vi "FindSectorBox.vi"(6 "reduce pts by factor of":i32=4, 7 "Sector EndPts":T5 {"y4" format="%.2f"; "x4" format="%.2f"; "y3" format="%.2f"; "x3" format="%.2f"; "y2" format="%.2f"; "x2" format="%.2f"; "y1" format="%.2f"; "x1" format="%.2f"}, 8 "sector size":cluster{"pixels in x":i16, "pixels in y":i16}={"pixels in x"=500, "pixels in y"=400}, 9 "directory path":path, 10 "File Array":string[](array[string]), 11 "File Index":i32) -> (0 "Fit Array":cluster{i32, i32, dbl, i32} {"?" format="%.2f"}, 1 "ROI (PramImage Subset co-ords)":T2 {"Subset TPI offset" format="%.2f"; "#TPI pts" format="%.2f"; "TPI start" format="%.2f"}, 2 "Subset dimensions":T4={"x start"=64, "x length"=1, "y start"=306, "y length"=318}, 3 "raw sector out":dbl[][](array[numeric]) format="%.2f", 4 "A/D bits":u16, 5 "Axis scaling Params":T1 {"Y high" format="%.2f"; "Y low" format="%.2f"; "X left" format="%.2f"; "X right" format="%.2f"})   [LabVIEW 2022 SP3]
panel:
  in  "Case Constant\n(See Context Help)":bool
  out "ROI in raw data co-ords":i16[][](graph)
  out "Region of Interest (raw co-ords)":T3 {"# rf pts" format="%.2f"; "start rf line" format="%.2f"; "start rf pt" format="%.2f"}
  out "Right side raw ROI":dbl[][](array[numeric]) format="%.2f"
  out "Left side raw ROI":dbl[][](array[numeric]) format="%.2f"
  out "top bottom of ROI":dbl[][](graph)
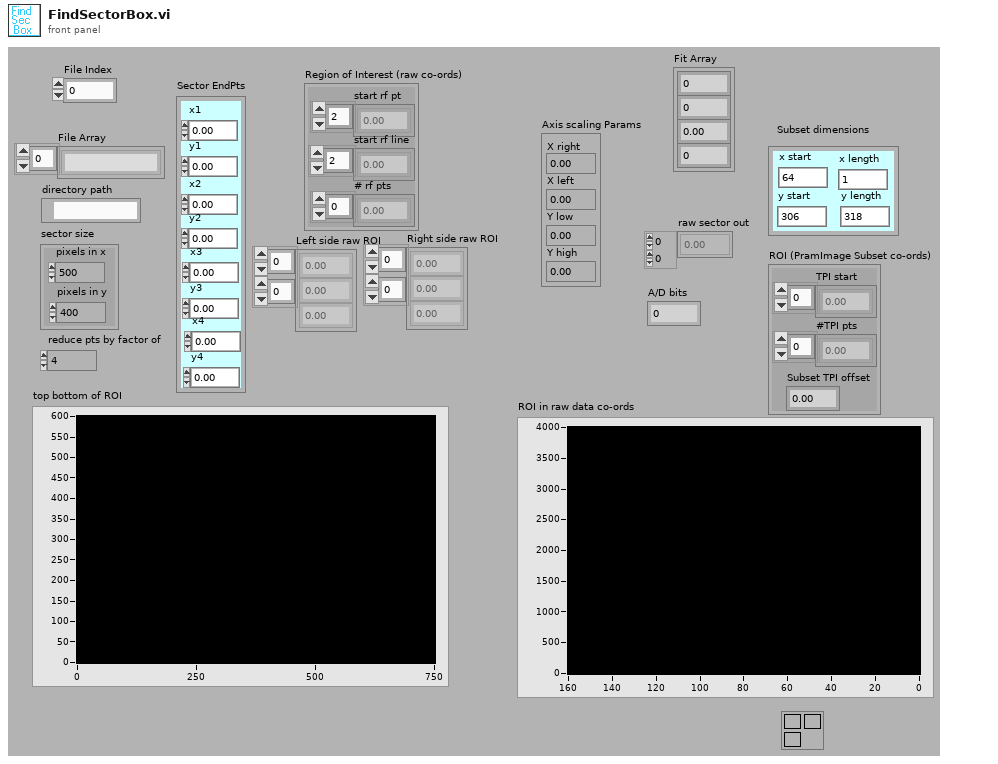
[diagram p1: front panel]
types:
  T1 = cluster{"X right":dbl, "X left":dbl, "Y low":dbl, "Y high":dbl}
  T2 = cluster{"TPI start":dbl[], "#TPI pts":dbl[], "Subset TPI offset":dbl}
  T3 = cluster{"start rf pt":dbl[], "start rf line":dbl[], "# rf pts":dbl[]}
  T4 = cluster{"x start":i32, "x length":i32, "y start":i32, "y length":i32}
  T5 = cluster{"x1":dbl, "y1":dbl, "x2":dbl, "y2":dbl, "x3":dbl, "y3":dbl, "x4":dbl, "y4":dbl}
  T6 = typedef "Header.ctl" = cluster{"header info":cluster{"Header":string, "Head length":i16}, "A/D info":cluster{"# rf points per line":u16, "# lines per scan":u16, "sample rate MHz":u16, "# A/D bits":i16, "# bytes per A/D":u16, "TGC Flag":u16, "A/D Type":string}, "Tranducer Info":cluster{"bandwidth":sgl, "center freq":sgl, "start freq":sgl, "ID":i32}, "Scan Info":cluster{"delay":sgl, "pivot distance":sgl, "sector scan angle":sgl, "operator":string, "Scan Mode":string, "location":string}, "Time/Date Info":cluster{"date":string, "time":string}, "RF Info":cluster{"RF file name":string, "RF file att":string, "RF cal file name":string, "RF cal file att":string}, "Patient Info":cluster{"ID":string, "extended ID":string, "age":u16, "sex":string, "previously\nscanned":string, "PSA":sgl, "LOS":u8, "Ethnicty 2":u8, "Race":u8}, "Tissue Type":cluster{"organ":i16, "disease type":i16, "disease location":i16}, "Votage scaling":cluster{"Digitizer (dB)":sgl, "Gain (dB)":sgl, "Atten (dB)":sgl}, "Comment":string, "Misc Info":cluster{"avg num":i16, "c speed":i16, "Div By or SF zones":i16, "XMIT CHS":u8, "RCV CHS":u8}, "Therapy Parameters":cluster{"Theraputic Freq (MHz)":sgl, "Time on (s)":sgl, "Therapy amplitude (mV)":sgl, "Lines Before":u16, "Lines After":u16}, "Scan Settings":cluster{"Energy (uJ or V)":u8, "Damp (Ohm) or Fc":u8, "HP Filt (KHz)":u8, "LP Filt (MHz)":u8, "Gain (db)":u8, "prf (kHz)":sgl, "Distance between\nscan lines (mm)":u16, "Distance between\nscan planes (mm)":u16}, "Compression Parameters":cluster{"F1 (MHz)":sgl, "F2 (MHz)":sgl, "% taper":sgl, "duration":sgl}, "Patient Info Xtra":cluster{"First Name":string, "Last Name":string, "Notes":string}}
  T7 = cluster{"delay":sgl, "pivot distance":sgl, "sector scan angle":sgl, "operator":string, "Scan Mode":string, "location":string}
  T8 = cluster{"y3":dbl, "x3":dbl, "y4":dbl, "x4":dbl, "x4":dbl, "x4":dbl, "x4":dbl, "x4":dbl}
  T9 = cluster{"y1":dbl, "x1":dbl, "y2":dbl, "x2":dbl, "x2":dbl, "x2":dbl, "x2":dbl, "x2":dbl}
  T10 = cluster{"x1":dbl, "y1":dbl, "x2":dbl, "y2":dbl, "x3":dbl, "y3":dbl, "x4":dbl, "y4":dbl}[]
  T11 = cluster{"y1":dbl, "x1":dbl, "y2":dbl, "x2":dbl, "x2":dbl, "x2":dbl, "x2":dbl, "x2":dbl}[]
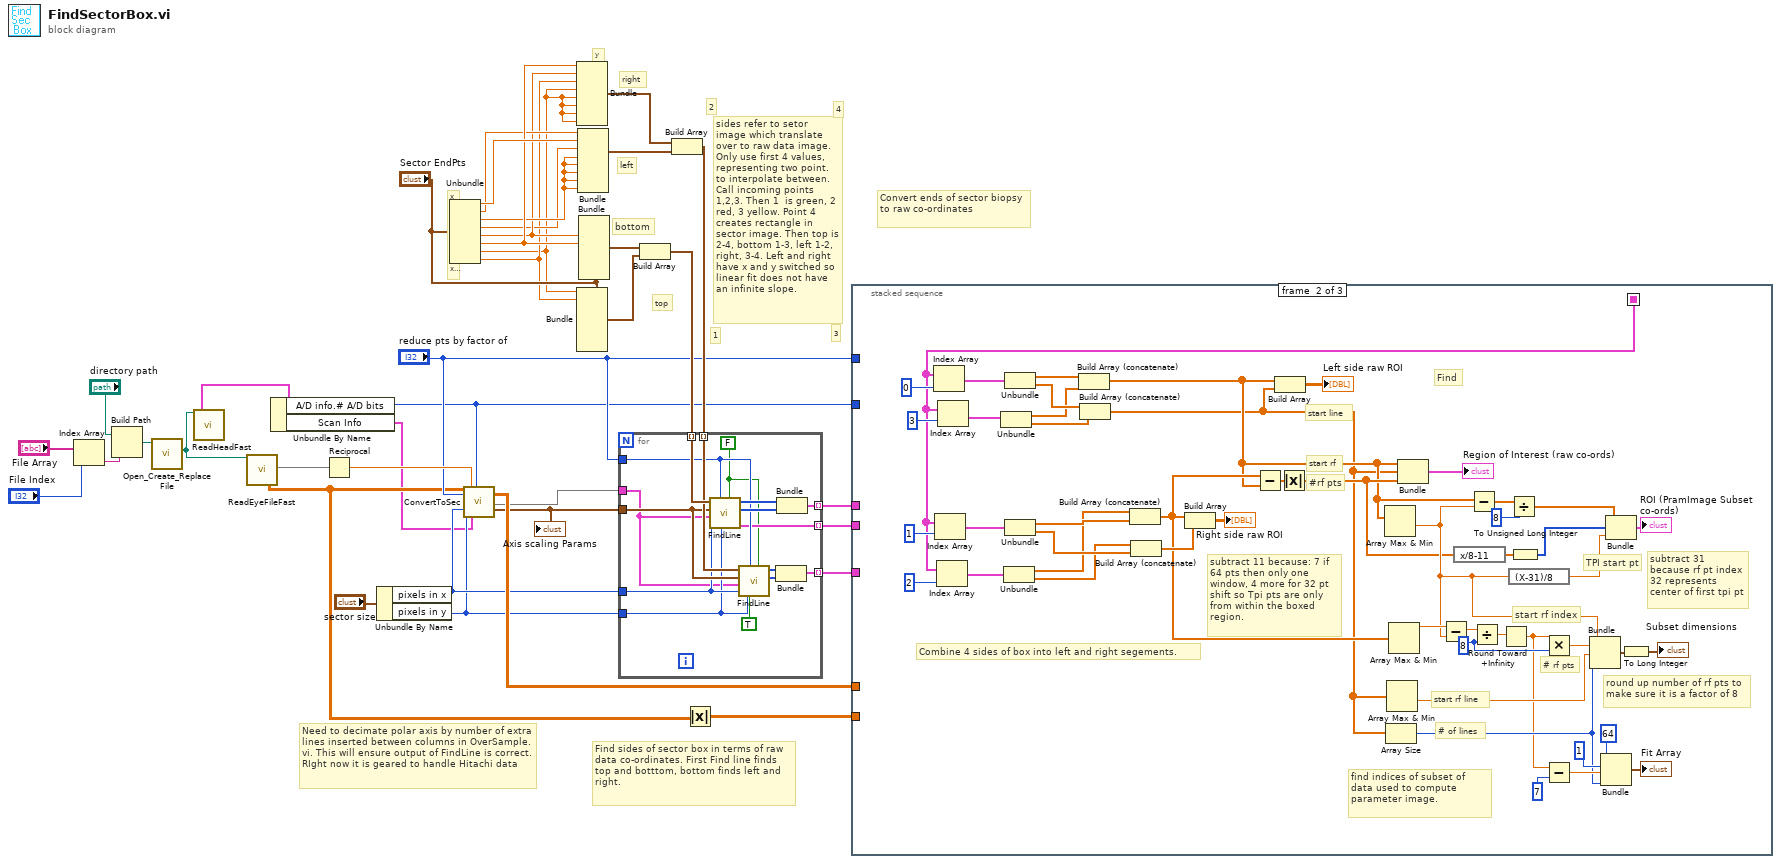
[diagram p0: block diagram]
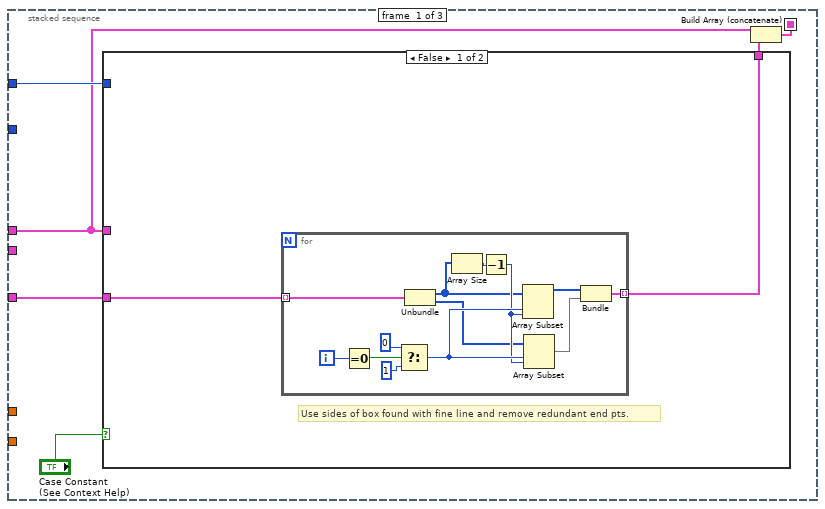
[diagram p2: hidden frame]
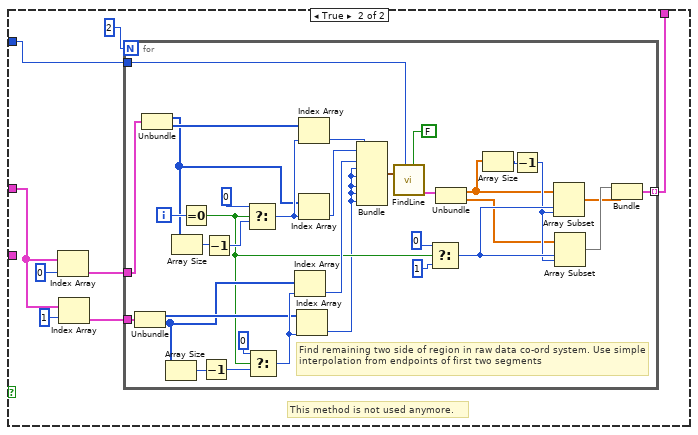
[diagram p3: hidden frame]
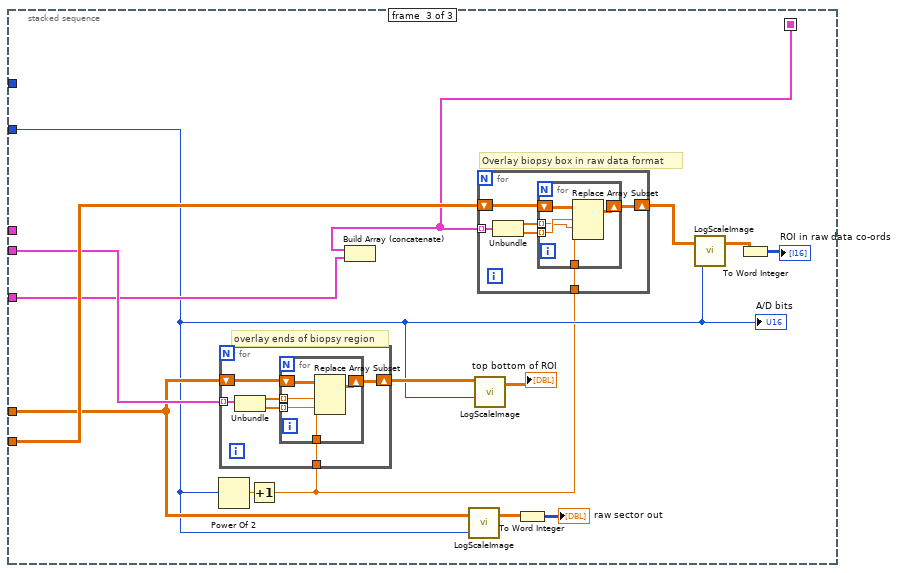
[diagram p4: hidden frame]
diagram:
  # "x4\ny4\nx2\ny2"
  # "x1\ny1\nx3\ny3"
  # "y1\nx1\ny2\nx2"
  # "y3\nx3\ny4\nx4"
  # "x1\ny1\nx2\ny2\nx3\ny3\nx4\ny4"
  # "4"
  # "3"
  # "2"
  # "1"
  # "sides refer to setor image which translate over to raw data image. Only use first 4 values, representing two point. to interpolate between. Call incoming points 1,2,3. Then 1  is green, 2 red, 3 yellow. Point 4 creates rectangle in sector image. Then top is 2-4, bottom 1-3, left 1-2, right, 3-4. Left and right have x and y switched so linear fit does not have an infinite slope."
  # "right"
  # "left"
  # "top"
  # "bottom"
  # "Need to decimate polar axis by number of extra lines inserted between columns in OverSample.vi. This will ensure output of FindLine is correct. RIght now it is geared to handle Hitachi data"
  # "Find sides of sector box in terms of raw data co-ordinates. First Find line finds top and botttom, bottom finds left and right."
  # "Convert ends of sector biopsy to raw co-ordinates"
  n1 = Index Array(array="File Array", index="File Index") -> (element=w38:string)
  n2 = Build Path(base path="directory path", name or relative path=w38) -> (appended path=w37:path)
  n3 = call <vilib>:"Open_Create_Replace File.vi"("file path"=w37) -> ("new file path"=w33:path)  [unwired: 5 in, 5 out]
  n4 = call "ReadHeadFast.vi"("new file path"=w33) -> ("Header In"=w2:T6)  [unwired: 15 in, 3 out]
  n5 = call "ReadEyeFileFast.vi"("new file path"=w33) -> ("2-D data array"=w3:sgl[][], 16:w34)  [unwired: 12 in, 5 out]
  n6 = Unbundle By Name(w2) -> ("A/D info.# A/D bits"=w4:i16, "Scan Info"=w1:T7)
  n7 = Reciprocal(x=w34) -> (1/x=w13:dbl)
  n8 = Unbundle By Name("sector size") -> ("pixels in x"=w25:i16, "pixels in y"=w24:i16)
  n9 = Unbundle("Sector EndPts") -> ("x1"=w20:dbl, "y1"=w18:dbl, "x2"=w10:dbl, "y2"=w7:dbl, "x3"=w8:dbl, "y3"=w19:dbl, "x4"=w5:dbl, "y4"=w6:dbl)
  n10 = call "ConvertToSec.vi"("raw image data in"=w3, "reduce pts by factor of"="reduce pts by factor of", "pixels in x"=w25, "pixels in y"=w24, "Time between rf pts\nmicros"=w13, "Scan Info"=w1, "Abs?"=w4) -> ("raw sector out"=w27:dbl[][], 17:w14, "Axis scaling Params"=w17:T1)  [unwired: 4 in, 6 out]
  "Axis scaling Params" <- w17
  n11 = Bundle("y3"=w19, "x3"=w8, "y4"=w6, "x4"=w5, "x4"=w5, "x4"=w5, "x4"=w5, "x4"=w5) -> (w9:T8)  [unwired: 1 out]
  n12 = Bundle(cluster="Sector EndPts", "x1"=w5, "y1"=w6) -> (w30:T5)  [unwired: 6 out]
  n13 = Bundle("y1"=w18, "x1"=w20, "y2"=w7, "x2"=w10, "x2"=w10, "x2"=w10, "x2"=w10, "x2"=w10) -> (w16:T9)  [unwired: 1 out]
  n14 = Bundle(cluster="Sector EndPts", "x2"=w8, "y2"=w19) -> (w22:T5)  [unwired: 6 out]
  n15 = Build Array(w22, w30) -> (w32:T10)
  n16 = Build Array(w9, w16) -> (w15:T11)
  n17 = for {
    tunnel: w17 -> [w46]
    tunnel: w14 -> [w42]
    tunnel: w25 -> [w45]
    tunnel: w24 -> [w44]
    tunnel: "reduce pts by factor of" -> [w43]
    tunnel: w32 -> [w51] mode=indexing
    tunnel: [w41] -> w31 mode=indexing
    tunnel: [w53] -> w29 mode=indexing
    tunnel: [w50] -> w23 mode=indexing
    tunnel: w15 -> [w47] mode=indexing
    w39 = FALSE
    n18 = call "FindLine.vi"("Box?"=w39, "pixels in y"=w44, "reduce pts by factor of"=w43, "pixels in x"=w45, "polar axis"=w42, "Axis scaling Params"=w46, "Sector EndPts"=w51) -> ("sector image line indices"=w41:cluster{"x indices":dbl[], "y indices":dbl[]}, "y indices"=w52:i32[], "x indices"=w54:i32[])  [unwired: 1 in, 1 out]
    n19 = call "FindLine.vi"("flip interp?"=TRUE, "Box?"=w39, "pixels in y"=w44, "reduce pts by factor of"=w43, "pixels in x"=w45, "polar axis"=w42, "Axis scaling Params"=w46, "Sector EndPts"=w47) -> ("y indices"=w48:i32[], "x indices"=w49:i32[])  [unwired: 2 out]
    n20 = Bundle("x indices"=w49, "y indices"=w48) -> (w50:cluster{"x indices":i32[], "y indices":i32[]})  [unwired: 1 out]
    n21 = Bundle("x indices"=w54, "y indices"=w52) -> (w53:cluster{"x indices":i32[], "y indices":i32[]})  [unwired: 1 out]
  }
  n22 = Absolute Value(x=w3) -> (abs(x)=w28:sgl[][])
  n23 = stacked-sequence {
    seq-local: [w59 _ _] -> [_ w142 w172]
    tunnel: w31 -> [_ _ w174]
    tunnel: w27 -> [_ _ w171]
    tunnel: "reduce pts by factor of" -> [w60 _ _]
    tunnel: w29 -> [w57 _ _]
    tunnel: w28 -> [_ _ w181]
    tunnel: w4 -> [_ _ w169]
    tunnel: w23 -> [w56 _ w173]
    frame #0 {
      n24 = case shown="False" "Case Constant\n(See Context Help)" {
        tunnel: w60 -> [_ w83]
        tunnel: [w61 w77] -> w58
        tunnel: w57 -> [_ w76]
        tunnel: w56 -> [w62 _]
        frame False {
          # "Use sides of box found with fine line and remove redundant end pts."
          n25 = for {
            tunnel: [w74] -> w61 mode=indexing
            tunnel: w62 -> [w65] mode=indexing
            i -> [w75]
            n26 = Equal To 0?(x=w75) -> (x = 0?=w66:bool)
            n27 = Select(t=0, s=w66, f=1) -> (s? t:f=w70:i32)
            n28 = Unbundle(w65) -> ("x indices"=w67:i32[], "y indices"=w68:i32[])
            n29 = Array Size(array=w67) -> (size(s)=w73:i32)
            n30 = Decrement(x=w73) -> (x-1=w69:i32)
            n31 = Array Subset(array=w67, index=w70, length=w69) -> (w64:i32[])
            n32 = Array Subset(array=w68, index=w70, length=w69) -> (w63:i32[])
            n33 = Bundle(w64, w63) -> (w74:cluster{i32[], i32[]})  [unwired: 1 out]
          }
        }
        frame True {
          # "This method is not used anymore."
          n34 = Index Array(array=w76, index=0) -> (element=w81:cluster{"x indices":i32[], "y indices":i32[]})
          n35 = Index Array(array=w76, index=1) -> (element=w80:cluster{"x indices":i32[], "y indices":i32[]})
          n36 = for {
            N: 2 -> [_]
            tunnel: w83 -> [w115]
            tunnel: w81 -> [w108]
            tunnel: w80 -> [w107]
            tunnel: [w95] -> w77 mode=indexing
            i -> [w117]
            # "Find remaining two side of region in raw data co-ord system. Use simple interpolation from endpoints of first two segments"
            n37 = Unbundle(w107) -> ("x indices"=w104:i32[], "y indices"=w103:i32[])
            n38 = Unbundle(w108) -> ("x indices"=w105:i32[], "y indices"=w106:i32[])
            n39 = Array Size(array=w103) -> (size(s)=w100:i32)
            n40 = Array Size(array=w105) -> (size(s)=w98:i32)
            n41 = Equal To 0?(x=w117) -> (x = 0?=w93:bool)
            n42 = Decrement(x=w100) -> (x-1=w99:i32)
            n43 = Decrement(x=w98) -> (x-1=w97:i32)
            n44 = Select(t=0, s=w93, f=w97) -> (s? t:f=w113:i32)
            n45 = Select(t=0, s=w93, f=w99) -> (s? t:f=w111:i32)
            n46 = Index Array(array=w103, index=w111) -> (element=w101:i32)
            n47 = Index Array(array=w104, index=w111) -> (element=w84:i32)
            n48 = Index Array(array=w106, index=w113) -> (element=w102:i32)
            n49 = Index Array(array=w105, index=w113) -> (element=w110:i32)
            n50 = Bundle(w102, w110, w101, w84, w84, w84, w84, w84) -> (w109:cluster{i32, i32, i32, i32, i32, i32, i32, i32})  [unwired: 1 out]
            n51 = call "FindLine.vi"("Box?"=FALSE, "reduce pts by factor of"=w115, "Sector EndPts"=w109) -> ("sector image line indices"=w96:cluster{"x indices":dbl[], "y indices":dbl[]})  [unwired: 5 in, 3 out]
            n52 = Select(t=0, s=w93, f=1) -> (s? t:f=w90:i32)
            n53 = Unbundle(w96) -> ("x indices"=w87:dbl[], "y indices"=w88:dbl[])
            n54 = Array Size(array=w87) -> (size(s)=w94:i32)
            n55 = Decrement(x=w94) -> (x-1=w89:i32)
            n56 = Array Subset(array=w87, index=w90, length=w89) -> (w85:dbl[])
            n57 = Array Subset(array=w88, index=w90, length=w89) -> (w86:dbl[])
            n58 = Bundle(w86, w85) -> (w95:cluster{dbl[], dbl[]})  [unwired: 1 out]
          }
        }
      }
      n59 = Build Array (concatenate)(w57, w58) -> (w59:cluster{"x indices":dbl[], "y indices":dbl[]}[])
    }
    frame #1 {
      w129 = 8
      # "round up number of rf pts to make sure it is a factor of 8"
      # "subtract 31 because rf pt index 32 represents center of first tpi pt"
      # "subtract 11 because: 7 if 64 pts then only one window, 4 more for 32 pt shift so Tpi pts are only from within the boxed region."
      # "TPI start pt"
      # "# of lines"
      # "start rf line"
      # "# rf pts"
      # "start rf index"
      # "Find"
      # "Combine 4 sides of box into left and right segements."
      # "find indices of subset of data used to compute parameter image."
      # "#rf pts"
      # "start rf"
      # "start line"
      n60 = Index Array(array=w142, index=0) -> (element=w162:cluster{"x indices":dbl[], "y indices":dbl[]})
      n61 = Index Array(array=w142, index=1) -> (element=w159:cluster{"x indices":dbl[], "y indices":dbl[]})
      n62 = Index Array(array=w142, index=2) -> (element=w160:cluster{"x indices":dbl[], "y indices":dbl[]})
      n63 = Index Array(array=w142, index=3) -> (element=w161:cluster{"x indices":dbl[], "y indices":dbl[]})
      n64 = Unbundle(w161) -> ("x indices"=w141:dbl[], "y indices"=w140:dbl[])
      n65 = Unbundle(w160) -> ("x indices"=w139:dbl[], "y indices"=w138:dbl[])
      n66 = Unbundle(w162) -> ("x indices"=w158:dbl[], "y indices"=w157:dbl[])
      n67 = Unbundle(w159) -> ("x indices"=w156:dbl[], "y indices"=w155:dbl[])
      n68 = Build Array (concatenate)(w158, w141) -> (w121:dbl[])
      n69 = Build Array (concatenate)(w157, w140) -> (w120:dbl[])
      n70 = Build Array (concatenate)(w139, w156) -> (w132:dbl[])
      n71 = Build Array (concatenate)(w138, w155) -> (w154:dbl[])
      n72 = Build Array(w132, w154) -> (→"Right side raw ROI":dbl[][])
      n73 = Subtract(x=w132, y=w121) -> (x-y=w133:dbl[])
      n74 = Build Array(w121, w120) -> (→"Left side raw ROI":dbl[][])
      n75 = Absolute Value(x=w133) -> (abs(x)=w123:dbl[])
      n76 = Array Max & Min(array=w121) -> (min value=w125:dbl)  [unwired: 3 out]
      n77 = Array Size(array=w120) -> (size(s)=w137:i32)
      n78 = Array Max & Min(array=w120) -> (min value=w144:dbl)  [unwired: 3 out]
      n79 = Array Max & Min(array=w132) -> (max value=w131:dbl)  [unwired: 3 out]
      n80 = Bundle(w121, w120, w123) -> (→"Region of Interest (raw co-ords)":cluster{dbl[], dbl[], dbl[]})  [unwired: 1 out]
      n81 = Subtract(x=w131, y=w125) -> (x-y=w130:dbl)
      n82 = expression code="x/8-11"(w123) -> (w122:dbl[])
      n83 = Subtract(x=w121, y=w125) -> (x-y=w134:dbl[])
      n84 = Divide(x=w130, y=w129) -> (x/y=w128:dbl)
      n85 = Round Toward +Infinity(x=w128) -> (ceil(x): smallest int >= x=w127:dbl)
      n86 = Divide(x=w134, y=8) -> (x/y=w135:dbl[])
      n87 = expression code="(X-31)/8"(w125) -> (w124:dbl)
      n88 = To Unsigned Long Integer(number=w122) -> (unsigned 32bit integer=w143:u32[])
      n89 = Multiply(x=w127, y=w129) -> (x*y=w149:dbl)
      n90 = Subtract(x=w127, y=7) -> (x-y=w147:dbl)
      n91 = Bundle(w125, w149, w144, w137) -> (w152:cluster{dbl, dbl, dbl, i32})  [unwired: 1 out]
      n92 = Bundle(64, 1, w147, w137) -> (→"Fit Array":cluster{i32, i32, dbl, i32})  [unwired: 1 out]
      n93 = Bundle(w135, w143, w124) -> (→"ROI (PramImage Subset co-ords)":cluster{dbl[], u32[], dbl})  [unwired: 1 out]
      n94 = To Long Integer(number=w152) -> (32bit integer=→"Subset dimensions":cluster{i32, i32, i32, i32})
    }
    frame #2 {
      # "Overlay biopsy box in raw data format"
      # "overlay ends of biopsy region"
      n95 = Power Of 2(x=w169) -> (2^x=w168:dbl)
      n96 = Increment(x=w168) -> (x+1=w167:dbl)
      n97 = for {
        tunnel: w174 -> [w198] mode=indexing
        tunnel: w167 -> [w195]
        shift-right: [w193] -> w178
        shift-left: w171 -> [w194]
        n98 = Unbundle(w198) -> ("x indices"=w197:dbl[], "y indices"=w196:dbl[])
        n99 = for {
          shift-right: [w199] -> w193
          shift-left: w194 -> [w203]
          tunnel: w197 -> [w202] mode=indexing
          tunnel: w196 -> [w201] mode=indexing
          tunnel: w195 -> [w200]
          n100 = Replace Array Subset(array=w203, new element=w200, index (row)=w202, index (col)=w201) -> (w199:dbl[][])
        }
      }
      n101 = Build Array (concatenate)(w172, w173) -> ()  [unwired: 1 out]
      n102 = call "LogScaleImage.vi"("A/D bits"=w169, "input array"=w171) -> ("log scale image"=w180:dbl[][])  [unwired: 1 out]
      n103 = call "LogScaleImage.vi"("A/D bits"=w169, "input array"=w178) -> ("log scale image"=→"top bottom of ROI":dbl[][])  [unwired: 1 out]
      n104 = for {
        tunnel: w167 -> [w185]
        shift-right: [w183] -> w177
        shift-left: w181 -> [w184]
        tunnel: w172 -> [w182] mode=indexing
        n105 = Unbundle(w182) -> ("x indices"=w187:dbl[], "y indices"=w186:dbl[])
        n106 = for {
          shift-right: [w191] -> w183
          shift-left: w184 -> [w192]
          tunnel: w187 -> [w188] mode=indexing
          tunnel: w186 -> [w189] mode=indexing
          tunnel: w185 -> [w190]
          n107 = Replace Array Subset(array=w192, new element=w190, index (row)=w189, index (col)=w188) -> (w191:sgl[][])
        }
      }
      n108 = To Word Integer(number=w180) -> (16bit integer=→"raw sector out":i16[][])
      n109 = call "LogScaleImage.vi"("A/D bits"=w169, "input array"=w177) -> ("log scale image"=w176:dbl[][])  [unwired: 1 out]
      n110 = To Word Integer(number=w176) -> (16bit integer=→"ROI in raw data co-ords":i16[][])
      "A/D bits" <- w169
    }
  }
